vi "Resize Icons.vi"(10 "Scale Factor":dbl=0.75, 11 "Filtered Command Info Out":T1) -> (3 "Filtered Command Info Out":T1)   [LabVIEW 2023]
uses:
  Types/Command Editor Info.ctl
  Types/Single Cmd Info.ctl
  <vilib>/picture/picture.llb/imagedata.ctl
  <vilib>/vision/NI_Vision_Development_Module.lvlib
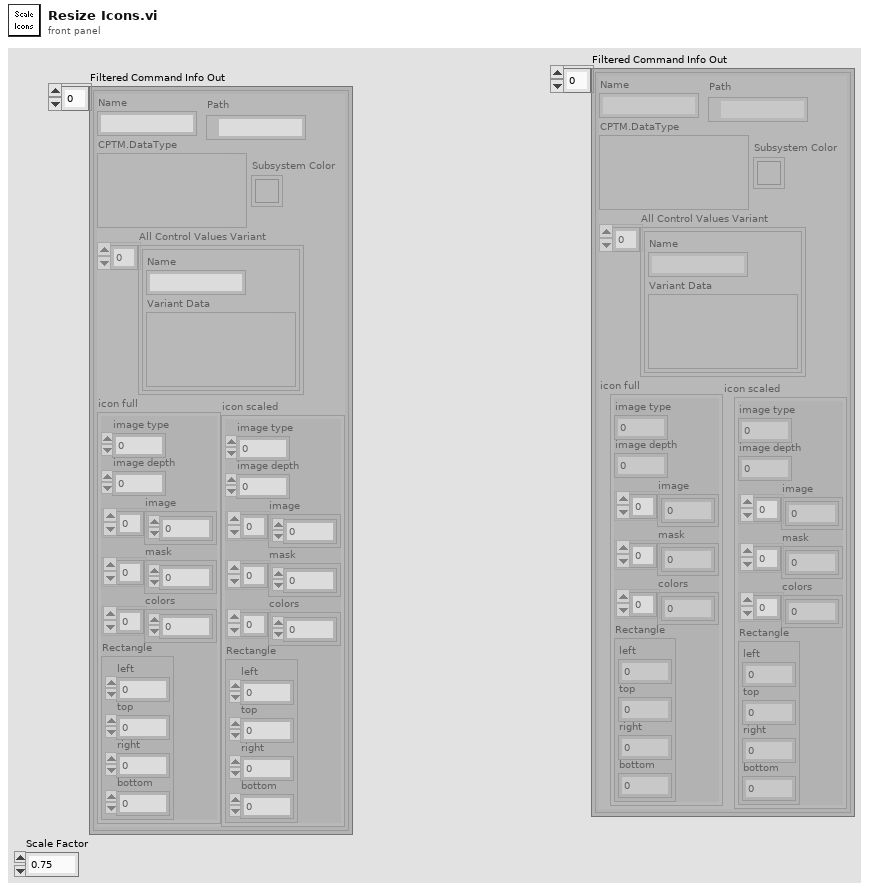
[diagram p1: front panel]
types:
  T1 = typedef "Command Editor Info.ctl" = T2[]
  T2 = typedef "Single Cmd Info.ctl" = cluster{"Name":string, "CPTM.DataType":variant, "All Control Values Variant":cluster{"Name":string, "Variant Data":variant}[], "icon full":T3, "icon scaled":T3, "Path":path, "Subsystem Color":u32}
  T3 = typedef "imagedata.ctl" = cluster{"image type":i32, "image depth":i32, "image":u8[], "mask":u8[], "colors":u32[], "Rectangle":cluster{"left":i16, "top":i16, "right":i16, "bottom":i16}}
  T4 = typedef "Image Type" = u32
  T5 = cluster{"left":i16, "top":i16, "right":i16, "bottom":i16}
  T6 = typedef "IMAQ Image.ctl" = refnum<image>
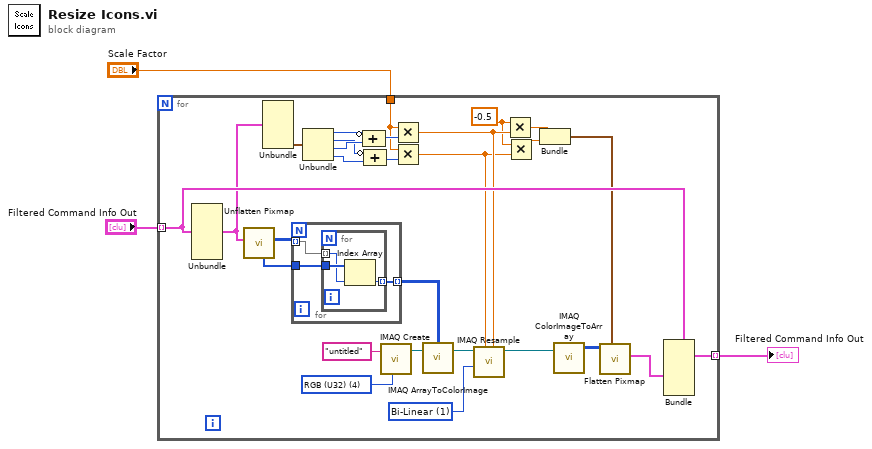
[diagram p0: block diagram]
diagram:
  n1 = for {
    tunnel: "Filtered Command Info Out" -> [w12] mode=indexing
    tunnel: [w11] -> w2 mode=indexing
    tunnel: "Scale Factor" -> [w14]
    w7 = -0.5
    w26 = u32 1 items=["Zero Order", "Bi-Linear", "Quadratic", "Cubic Spline"] ("Interpolation Type")
    w28 = T4 4 items=["Grayscale (U8)", "Grayscale (I16)", "Grayscale (SGL)", "Complex (CSG)", "RGB (U32)", "HSL (U32)", "RGB (U64)", "Grayscale (U16)"] ("Image Type")
    n2 = Unbundle(w12) -> ("icon full"=w10:T3)  [unwired: 6 out]
    n3 = call <vilib>:"Unflatten Pixmap.vi"("image data"=w10) -> ("8-bit pixmap"=w25:u8[][], "colors"=w24:u32[])  [unwired: 4 in, 5 out]
    n4 = Unbundle(w10) -> ("Rectangle"=w20:T5)  [unwired: 5 out]
    n5 = for {
      tunnel: w25 -> [w34] mode=indexing
      tunnel: w24 -> [w33]
      tunnel: [w32] -> w23 mode=indexing
      n6 = for {
        tunnel: w34 -> [w36] mode=indexing
        tunnel: w33 -> [w37]
        tunnel: [w35] -> w32 mode=indexing
        n7 = Index Array(array=w37, index=w36) -> (element=w35:u32)
      }
    }
    n8 = Unbundle(w20) -> ("left"=w19:i16, "top"=w16:i16, "right"=w18:i16, "bottom"=w15:i16)
    n9 = Compound Arithmetic op=ADD(invert w19, w18) -> (w17:i16)
    n10 = Compound Arithmetic op=ADD(invert w16, w15) -> (w13:i16)
    n11 = call "IMAQ Create"("Image Name"="untitled", "Image Type"=w28) -> ("New Image"=w29:T6)  [unwired: 3 in, 1 out]
    n12 = Multiply(x=w14, y=w17) -> (x*y=w9:dbl)
    n13 = Multiply(x=w14, y=w13) -> (x*y=w6:dbl)
    n14 = call "IMAQ ArrayToColorImage"("Image Pixels (U32)"=w23, "Image"=w29) -> ("Image Out"=w31:T6)  [unwired: 3 in, 1 out]
    n15 = call "IMAQ Resample"("X Resolution"=w9, "Y Resolution"=w6, "Interpolation Type"=w26, "Image Src"=w31) -> ("Image Dst Out"=w30:T6)  [unwired: 6 in, 1 out]
    n16 = Multiply(x=w7, y=w9) -> (x*y=w8:dbl)
    n17 = Multiply(x=w7, y=w6) -> (x*y=w5:dbl)
    n18 = Bundle(w8, w5) -> (w4:cluster{dbl, dbl})  [unwired: 1 in]
    n19 = call "IMAQ ColorImageToArray"("Image"=w30) -> ("Image Pixels (U32)"=w22:u32[][])  [unwired: 3 in, 2 out]
    n20 = call <vilib>:"Flatten Pixmap.vi"("top left"=w4, "24-bit pixmap"=w22) -> ("image data"=w21:T3)  [unwired: 9 in]
    n21 = Bundle(cluster=w12, "icon scaled"=w21) -> (w11:T2)  [unwired: 6 in]
  }
  "Filtered Command Info Out" <- w2
